vi "Dvmg Get Dev Name.vi"(8 "error in (no error)":errorcluster, 9 "perc":i32, 10 "szdvcTemp":string, 11 "idvc":i32) -> (0 "error out":errorcluster, 1 "perc out":i32, 2 "szdvcTemp out":string, 3 "function return":i32)   [LabVIEW 2011, in "LVH-Adept.lvlib" / "DPCUTIL.lvlib"]
doc: "DPCAPI BOOL DvmgGetDevName(INT32 idvc, char * szdvcTemp, ERC * perc);"
uses:
  DPCUTIL.lvlib
  <vilib>/LabVIEW Hacker/Adept/Private/Resources/dpcutil.dll
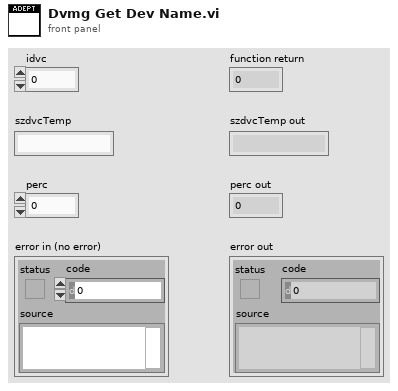
[diagram p1: front panel]
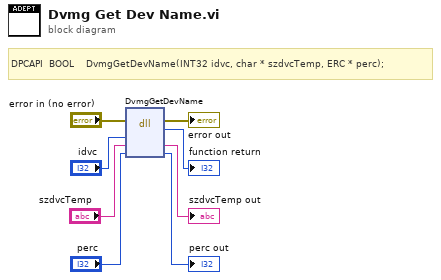
[diagram p0: block diagram]
diagram:
  # "DPCAPI  BOOL    DvmgGetDevName(INT32 idvc, char * szdvcTemp, ERC * perc);"
  n1 = dll-call lib="C:/Program Files (x86)/National Instruments/LabVIEW 2011/vi.lib/LabVIEW Hacker/Adept/Private/Resources/dpcutil.*" fn="DvmgGetDevName"(error in="error in (no error)", "idvc"="idvc", "szdvcTemp"="szdvcTemp", "perc"="perc") -> (error out=→"error out":errorcluster, →"function return":i32, "szdvcTemp"=→"szdvcTemp out":string, "perc"=→"perc out":i32)  [unwired: 3 in, 1 out]
